vi "LSMcontroller_v59_PIzstage.vi"() -> ()   [LabVIEW 2015] (continued)
                        n2597 = Unbundle By Name(w5609) -> ("AO parameters"=w5607:T25)
                        n2598 = Index Array(array=w5607, index=0) -> (element=w5606:T26)
                        n2599 = call "generateRampedSquareWave_fromAOparameters.vi"("AO params"=w5606) -> ("Waveform"=w5602:waveform(dbl), "wflength"=w5603:i32)
                        n2600 = Build Array(w5602) -> (w5605:waveform(dbl)[])
                        n2601 = call "waveformssealtestbuffer.vi"("AO wf in"=w5605, "command"="set") -> ()  [unwired: 1 out]
                      }
                      frame #2 {
                        n2602 = local read "Vholding (mV)"() -> (w5612:sgl)
                        n2603 = local read "Current Clamp"() -> (w5618:bool)
                        n2604 = local read "Voltage Clamp"() -> (w5617:bool)
                        n2605 = local read "OCgain"() -> (w5613:sgl)
                        n2606 = local read "CC_ICgain"() -> (w5616:dbl)
                        n2607 = local read "holdon"() -> (w5611:bool)
                        n2608 = call "patchparameters.vi"("command"="get") -> ("Params out"=w5620:T14)  [unwired: 1 in]
                        n2609 = Bundle By Name(cluster=w5620, "VC"=w5617, "CC"=w5618, "CC_icg (pA/mv)"=w5616, "VC_icg (mV/mV)"=10.0, "OCG (mV/pA)"=w5613, "OVG (mV/mV)"=0.1, "Vhold (mV)"=w5612, "holdon"=w5611) -> (w5619:T14)
                        n2610 = call "patchparameters.vi"("Params in"=w5619, "command"="set") -> ()  [unwired: 1 out]
                      }
                    }
                  }
                  frame #1 {
                    w5623 = 2
                    n2611 = call "patchparameters.vi"("command"="get") -> ("Params out"=w5631:T14)  [unwired: 1 in]
                    n2612 = Unbundle By Name(w5631) -> ("holdon"=w5630:bool, "Vhold (mV)"=w5629:sgl, "CC_icg (pA/mv)"=w5637:sgl, "CC"=w5635:bool, "VC_icg (mV/mV)"=w5636:sgl)
                    n2613 = Select(t=w5637, s=w5635, f=w5636) -> (s? t:f=w5638:sgl)
                    n2614 = To Single Precision Float(number=0.001 ("y")) -> (single precision float=w5639:sgl)
                    n2615 = Compound Arithmetic op=MULTIPLY(w5629, w5638, w5639) -> (w5633:sgl)
                    n2616 = case shown="False" w5630 {
                      tunnel: w5633 -> [_ w5651]
                      tunnel: [0.0 w5651] -> w5626
                      frame False {
                      }
                      frame True {
                      }
                    }
                    n2617 = Greater Than 0?(x=w5623) -> (x > 0?=w5625:bool)
                    n2618 = case shown="True" w5625 {
                      tunnel: w5624 -> [_ w5640]
                      tunnel: w5623 -> [_ w5643]
                      frame False {
                      }
                      frame True {
                        n2619 = Initialize Array(sgl 0.0 ("element"), w5643, w5640) -> (w5641:sgl[][])
                        n2620 = call "allAI-temp.vi"("array in"=w5641, "command"=enum16{"get", "set", "clear", "append"}."set") -> ()  [unwired: 2 in, 2 out]
                      }
                    }
                    n2621 = flat-sequence {
                      tunnel: w5624 -> [w5647]
                      tunnel: w5624 -> [w5646]
                      tunnel: [w5646] -> w5628
                      tunnel: [w5645] -> w5627
                      tunnel: w5626 -> [w5645]
                      tunnel: w5628 -> [w5649]
                      tunnel: w5627 -> [w5648]
                      frame #0 {
                        n2622 = call "prepAI_sealtest.vi"("samples per channel"=w5647) -> ()  [unwired: 2 in]
                      }
                      frame #1 {
                        n2623 = call "prepAO_sealtest.vi"("Vhold"=w5648, "samples per channel"=w5649) -> ()  [unwired: 1 in]
                      }
                    }
                  }
                  frame #2 {
                    n2624 = stacked-sequence {
                      frame #0 {
                        n2625 = call "tempconfigAO.vi"("command"="get") -> ("Temp Config out"=w5655:T27)  [unwired: 1 in]
                        n2626 = Unbundle By Name(w5655) -> ("AO"=w5656:refnum<k21>[], "E_AO"=w5657:errorcluster[])
                        n2627 = for {
                          tunnel: w5656 -> [w5665] mode=indexing
                          tunnel: w5657 -> [w5664] mode=indexing
                          tunnel: [w5663] -> w5659 mode=indexing
                          tunnel: [w5662] -> w5660 mode=indexing
                          n2628 = call <vilib>:"DAQmx Start Task.vi"("task/channels in"=w5665, "error in"=w5664) -> ("task out"=w5663:refnum<k21>, "error out"=w5662:errorcluster)  [unwired: 12 in]
                        }
                        n2629 = call "tempconfigAO.vi"("command"="get") -> ("Temp Config out"=w5658:T27)  [unwired: 1 in]
                        n2630 = Bundle By Name(cluster=w5658, "AO"=w5659, "E_AO"=w5660) -> (w5661:T27)
                        n2631 = call "tempconfigAO.vi"("Temp Config in"=w5661, "command"="set") -> ()  [unwired: 1 out]
                      }
                      frame #1 {
                        n2632 = call "tempconfigAI.vi"("command"="get") -> ("Temp Config out"=w5667:T28)  [unwired: 1 in]
                        n2633 = Unbundle By Name(w5667) -> ("AI"=w5672:refnum<k21>, "E_AI"=w5673:errorcluster)
                        n2634 = call <vilib>:"DAQmx Start Task.vi"("task/channels in"=w5672, "error in"=w5673) -> ("task out"=w5674:refnum<k21>, "error out"=w5675:errorcluster)  [unwired: 12 in]
                        n2635 = call "tempconfigAI.vi"("command"="get") -> ("Temp Config out"=w5669:T28)  [unwired: 1 in]
                        n2636 = Bundle By Name(cluster=w5669, "AI"=w5674, "E_AI"=w5675) -> (w5671:T28)
                        n2637 = call "tempconfigAI.vi"("Temp Config in"=w5671, "command"="set") -> ()  [unwired: 1 out]
                      }
                    }
                  }
                  frame #3 {
                    n2638 = while {
                      tunnel: w5676 -> [w5677]
                      stop <- w5678 stop-if-true
                      n2639 = local read "sealtest"() -> (w5681:bool)
                      n2640 = Not(x=w5681) -> (.not. x?=w5680:bool)
                      n2641 = case shown="False" w5680 {
                        tunnel: w5677 -> [w5682 _]
                        frame False {
                          n2642 = stacked-sequence {
                            seq-local: [_ _ _ w5721 _ _] -> [_ _ _ _ w5777 _]
                            seq-local: [w5683 _ _ _ _ _] -> [_ w5692 _ w5714 w5766 w5797]
                            tunnel: w5682 -> [_ _ w5700 _ w5765 _]
                            frame #0 {
                              n2643 = call "patchparameters.vi"("command"="get") -> ("Params out"=w5690:T14)  [unwired: 1 in]
                              n2644 = local read "Vholding (mV)"() -> (w5687:sgl)
                              n2645 = Unbundle By Name(w5690) -> ("Vhold (mV)"=w5686:sgl, "holdon"=w5689:bool)
                              n2646 = local read "holdon"() -> (w5688:bool)
                              n2647 = Not Equal?(x=w5687, y=w5686) -> (x != y?=w5685:bool)
                              n2648 = Not Equal?(x=w5689, y=w5688) -> (x != y?=w5684:bool)
                              n2649 = Or(x=w5685, y=w5684) -> (x .or. y?=w5683:bool)
                            }
                            frame #1 {
                              n2650 = case shown="True" w5692 {
                                frame False {
                                }
                                frame True {
                                n2651 = local read "Vholding (mV)"() -> (w5695:sgl)
                                n2652 = local read "holdon"() -> (w5693:bool)
                                n2653 = call "patchparameters.vi"("command"="get") -> ("Params out"=w5696:T14)  [unwired: 1 in]
                                n2654 = Bundle By Name(cluster=w5696, "Vhold (mV)"=w5695, "holdon"=w5693) -> (w5694:T14)
                                n2655 = call "patchparameters.vi"("Params in"=w5694, "command"="set") -> ()  [unwired: 1 out]
                                }
                              }
                            }
                            frame #2 {
                              n2656 = call "tempconfigAI.vi"("command"="get") -> ("Temp Config out"=w5710:T28)  [unwired: 1 in]
                              n2657 = Unbundle By Name(w5710) -> ("AI"=w5709:refnum<k21>, "E_AI"=w5708:errorcluster)
                              n2658 = call-poly <vilib>:"DAQmx Read.vi"("task/channels in"=w5709, "number of samples per channel"=w5700, "timeout"=10.0, "error in"=w5708) -> ("task out"=w5704:refnum<k21>, "data"=w5701:i16[][], "error out"=w5713:errorcluster)  [unwired: 9 in]
                              n2659 = call "tempconfigAI.vi"("command"="get") -> ("Temp Config out"=w5705:T28)  [unwired: 1 in]
                              n2660 = Bundle By Name(cluster=w5705, "AI"=w5704, "E_AI"=w5713) -> (w5712:T28)
                              n2661 = To Single Precision Float(number=w5701) -> (single precision float=w5703:sgl[][])
                              n2662 = call "tempconfigAI.vi"("Temp Config in"=w5712, "command"="set") -> ()  [unwired: 1 out]
                              n2663 = call "allAI-temp.vi"("array in"=w5703, "command"=enum16{"get", "set", "clear", "append"}."set") -> ()  [unwired: 2 in, 2 out]
                            }
                            frame #3 {
                              n2664 = case shown="True" w5714 {
                                frame False {
                                }
                                frame True {
                                n2665 = call "tempconfigAO.vi"("command"="get") -> ("Temp Config out"=w5754:T27)  [unwired: 1 in]
                                n2666 = Unbundle By Name(w5754) -> ("AO"=w5753:refnum<k21>[], "E_AO"=w5752:errorcluster[])
                                n2667 = call "tempconfigAI.vi"("command"="get") -> ("Temp Config out"=w5741:T28)  [unwired: 1 in]
                                n2668 = Unbundle By Name(w5741) -> ("AI"=w5742:refnum<k21>, "E_AI"=w5743:errorcluster)
                                n2669 = for {
                                tunnel: w5753 -> [w5758] mode=indexing
                                tunnel: w5752 -> [w5757] mode=indexing
                                tunnel: [w5756] -> w5748 mode=indexing
                                n2670 = call <vilib>:"DAQmx Stop Task.vi"("task/channels in"=w5758, "error in"=w5757) -> ("task out"=w5759:refnum<k21>, "error out"=w5760:errorcluster)  [unwired: 12 in]
                                n2671 = call <vilib>:"DAQmx Clear Task.vi"("task in"=w5759, "error in"=w5760) -> ("error out"=w5756:errorcluster)  [unwired: 13 in]
                                }
                                n2672 = call <vilib>:"DAQmx Stop Task.vi"("task/channels in"=w5742, "error in"=w5743) -> ("task out"=w5739:refnum<k21>, "error out"=w5738:errorcluster)  [unwired: 12 in]
                                n2673 = call <vilib>:"DAQmx Clear Task.vi"("task in"=w5739, "error in"=w5738) -> ("error out"=w5737:errorcluster)  [unwired: 13 in]
                                n2674 = call "tempconfigAO.vi"("command"="get") -> ("Temp Config out"=w5749:T27)  [unwired: 1 in]
                                n2675 = Bundle By Name(cluster=w5749, "E_AO"=w5748) -> (w5747:T27)
                                n2676 = call "tempconfigAI.vi"("command"="get") -> ("Temp Config out"=w5745:T28)  [unwired: 1 in]
                                n2677 = Bundle By Name(cluster=w5745, "E_AI"=w5737) -> (w5736:T28)
                                n2678 = call "tempconfigAO.vi"("Temp Config in"=w5747, "command"="set") -> ()  [unwired: 1 out]
                                n2679 = call "tempconfigAI.vi"("Temp Config in"=w5736, "command"="set") -> ()  [unwired: 1 out]
                                }
                              }
                              n2680 = call "allAI-temp.vi"("command"=enum16{"get", "set", "clear", "append"}."get") -> ("array out"=w5718:sgl[][])  [unwired: 3 in, 1 out]
                              n2681 = call "tempconfigAI.vi"("command"="get") -> ("Temp Config out"=w5731:T28)  [unwired: 1 in]
                              n2682 = call "tempconfigAI.vi"("command"="get") -> ("Temp Config out"=w5733:T28)  [unwired: 1 in]
                              n2683 = Unbundle By Name(w5731) -> ("header"=w5729:dbl[])
                              n2684 = Unbundle By Name(w5733) -> ("header"=w5735:dbl[])
                              n2685 = Index Array(array=w5718, index (row) #1=1 ("index (row)"), index (row) #2=0 ("index (row)")) -> (element #1=w5716:sgl[], element #2=w5715:sgl[])  [unwired: 2 in]
                              n2686 = local read "OCgain"() -> (w5723:sgl)
                              n2687 = call "Unscaledtoscaled.vi"("Unscaled Data"=w5716, "Header Information"=w5729) -> ("Array"=w5728:sgl[])  [unwired: 1 in]
                              n2688 = call "Unscaledtoscaled.vi"("Unscaled Data"=w5715, "Header Information"=w5735) -> ("Array"=w5732:sgl[])  [unwired: 1 in]
                              n2689 = Multiply(x=w5728, y=0.1) -> (x*y=w5725:dbl[])
                              n2690 = Divide(x=w5732, y=w5723) -> (x/y=w5724:sgl[])
                              n2691 = Build Array(w5725, w5724) -> (w5727:dbl[][])
                              n2692 = Multiply(x=w5727, y=1000.0) -> (x*y=w5721:dbl[][])
                              "Patch readout" <- w5721
                            }
                            frame #4 {
                              n2693 = case shown="True" w5766 {
                                tunnel: w5765 -> [_ w5778]
                                frame False {
                                }
                                frame True {
                                n2694 = call "patchparameters.vi"("command"="get") -> ("Params out"=w5782:T14)  [unwired: 1 in]
                                n2695 = Unbundle By Name(w5782) -> ("holdon"=w5781:bool, "Vhold (mV)"=w5780:sgl, "CC_icg (pA/mv)"=w5788:sgl, "CC"=w5786:bool, "VC_icg (mV/mV)"=w5787:sgl)
                                n2696 = Select(t=w5788, s=w5786, f=w5787) -> (s? t:f=w5789:sgl)
                                n2697 = To Single Precision Float(number=0.001 ("y")) -> (single precision float=w5790:sgl)
                                n2698 = Compound Arithmetic op=MULTIPLY(w5780, w5789, w5790) -> (w5784:sgl)
                                n2699 = case shown="True" w5781 {
                                tunnel: w5784 -> [_ w5795]
                                tunnel: [0.0 w5795] -> w5779
                                frame False {
                                }
                                frame True {
                                }
                                }
                                n2700 = flat-sequence {
                                tunnel: w5778 -> [w5791]
                                tunnel: w5779 -> [w5793]
                                tunnel: w5778 -> [w5792]
                                frame #0 {
                                n2701 = call "prepAI_sealtest.vi"("samples per channel"=w5791) -> ()  [unwired: 2 in]
                                }
                                frame #1 {
                                n2702 = call "prepAO_sealtest.vi"("Vhold"=w5793, "samples per channel"=w5792) -> ()  [unwired: 1 in]
                                }
                                }
                                }
                              }
                              n2703 = call "sealtestwfparams.vi"("command"="get") -> ("Params out"=w5771:T24)  [unwired: 6 in]
                              n2704 = Unbundle By Name(w5771) -> ("AO parameters"=w5772:T25)
                              n2705 = Index Array(array=w5772, index=0) -> (element=w5774:T26)
                              n2706 = Unbundle By Name(w5774) -> ("Cycles"=w5769:dbl, "Start amplitude (V)"=w5768:dbl, "Sampling frequency (Hz)"=w5767:dbl)
                              n2707 = local read "fitpoints"() -> (w5775:dbl)
                              n2708 = script code="V=data(1,:);\nI=data(2,:);\ntres=mean(V);\nspc=(nsamp./ncyc);\nV=V(spc+1:end-spc);\nI=I(spc+1:end-spc);\ndV=mean(V(V>tres))-mean(V(V<tres))\nIcyc=reshape(I,[spc ncyc-2]);\nIcyc=Icyc';\nIcyc=mean(Icyc,1);\ndIss=mean(Icyc(floor(spc*0.15):floor(spc/2)-2))-mean(Icyc(spc*0.65:spc-2))\nRm=dV*1e3/dIss;\n[maxi,ind]=max(Icyc);\nIfit=Icyc(ind+1:ind+1+points-1)-0.5*(mean(Icyc(floor(spc*0.15):floor(spc/2)-2))+mean(Icyc(spc*0.65:spc-2)))\nt=(3:points-1+3)./srate*1000;\nt=t';\nIfit=Ifit';\nc=fit(t,Ifit, 'exp1');\ncoeffs=coeffvalues(c);\nIa=coeffs(1);\nRa=dV*1e3./Ia/2;\ntau=-1./coeffs(2);\ncap=tau/Ra*1000;"("data"=w5777, "nsamp"=w5765, "ncyc"=w5769, "maxV"=w5768, "points"=w5775, "srate"=w5767) -> ("cap"=w5764:dbl, "Ra"=w5763:dbl, "Icyc"=w5762:dbl[], "Rm"=w5761:dbl)  [unwired: 1 in, 1 out]
                              n2709 = local read "set as Rp?"() -> (w5776:bool)
                              n2710 = local write "Cmembrane"(w5764) -> ()
                              n2711 = local write "Rmembrane (MOhm)"(w5761) -> ()
                              n2712 = local write "Racces (MOhm)"(w5763) -> ()
                              n2713 = case shown="True" w5776 {
                                tunnel: w5761 -> [_ w5796]
                                frame False {
                                }
                                frame True {
                                n2714 = local write "Rpipette (MOhm)"(w5796) -> ()
                                }
                              }
                              n2715 = local write "Ifit"(w5762) -> ()
                            }
                            frame #5 {
                              n2716 = local read "set as Rp?"() -> (w5798:bool)
                              n2717 = case shown="True" w5797 {
                                frame False {
                                }
                                frame True {
                                n2718 = stacked-sequence {
                                frame #0 {
                                n2719 = call "tempconfigAO.vi"("command"="get") -> ("Temp Config out"=w5805:T27)  [unwired: 1 in]
                                n2720 = Unbundle By Name(w5805) -> ("AO"=w5804:refnum<k21>[], "E_AO"=w5803:errorcluster[])
                                n2721 = for {
                                tunnel: w5804 -> [w5812] mode=indexing
                                tunnel: w5803 -> [w5811] mode=indexing
                                tunnel: [w5810] -> w5801 mode=indexing
                                tunnel: [w5809] -> w5800 mode=indexing
                                n2722 = call <vilib>:"DAQmx Start Task.vi"("task/channels in"=w5812, "error in"=w5811) -> ("task out"=w5810:refnum<k21>, "error out"=w5809:errorcluster)  [unwired: 12 in]
                                }
                                n2723 = call "tempconfigAO.vi"("command"="get") -> ("Temp Config out"=w5802:T27)  [unwired: 1 in]
                                n2724 = Bundle By Name(cluster=w5802, "AO"=w5801, "E_AO"=w5800) -> (w5799:T27)
                                n2725 = call "tempconfigAO.vi"("Temp Config in"=w5799, "command"="set") -> ()  [unwired: 1 out]
                                }
                                frame #1 {
                                n2726 = call "tempconfigAI.vi"("command"="get") -> ("Temp Config out"=w5814:T28)  [unwired: 1 in]
                                n2727 = Unbundle By Name(w5814) -> ("AI"=w5819:refnum<k21>, "E_AI"=w5820:errorcluster)
                                n2728 = call <vilib>:"DAQmx Start Task.vi"("task/channels in"=w5819, "error in"=w5820) -> ("task out"=w5821:refnum<k21>, "error out"=w5822:errorcluster)  [unwired: 12 in]
                                n2729 = call "tempconfigAI.vi"("command"="get") -> ("Temp Config out"=w5816:T28)  [unwired: 1 in]
                                n2730 = Bundle By Name(cluster=w5816, "AI"=w5821, "E_AI"=w5822) -> (w5818:T28)
                                n2731 = call "tempconfigAI.vi"("Temp Config in"=w5818, "command"="set") -> ()  [unwired: 1 out]
                                }
                                }
                                }
                              }
                              n2732 = case shown="True" w5798 {
                                frame False {
                                }
                                frame True {
                                n2733 = local write "set as Rp?"(FALSE ("set as Rp?")) -> ()
                                }
                              }
                            }
                          }
                        }
                        frame True {
                        }
                      }
                      n2734 = local read "sealtest"() -> (w5679:bool)
                      n2735 = Not(x=w5679) -> (.not. x?=w5678:bool)
                    }
                  }
                  frame #4 {
                    n2736 = call "tempconfigAO.vi"("command"="get") -> ("Temp Config out"=w5849:T27)  [unwired: 1 in]
                    n2737 = Unbundle By Name(w5849) -> ("AO"=w5848:refnum<k21>[], "E_AO"=w5847:errorcluster[])
                    n2738 = call "configuration.vi"("command"="get") -> ("config out"=w5830:T12)  [unwired: 2 in, 1 out]
                    n2739 = call "tempconfigAI.vi"("command"="get") -> ("Temp Config out"=w5836:T28)  [unwired: 1 in]
                    n2740 = Unbundle By Name(w5830) -> ("Device 1 sampleclock out"=w5827:tag, "Device 1 Starttrigger out"=w5826:tag)
                    n2741 = Unbundle By Name(w5836) -> ("AI"=w5837:refnum<k21>, "E_AI"=w5838:errorcluster)
                    n2742 = for {
                      tunnel: w5848 -> [w5853] mode=indexing
                      tunnel: w5847 -> [w5852] mode=indexing
                      tunnel: [w5851] -> w5843 mode=indexing
                      n2743 = call <vilib>:"DAQmx Stop Task.vi"("task/channels in"=w5853, "error in"=w5852) -> ("task out"=w5854:refnum<k21>, "error out"=w5855:errorcluster)  [unwired: 12 in]
                      n2744 = call <vilib>:"DAQmx Clear Task.vi"("task in"=w5854, "error in"=w5855) -> ("error out"=w5851:errorcluster)  [unwired: 13 in]
                    }
                    n2745 = call <vilib>:"DAQmx Stop Task.vi"("task/channels in"=w5837, "error in"=w5838) -> ("task out"=w5834:refnum<k21>, "error out"=w5833:errorcluster)  [unwired: 12 in]
                    n2746 = call <vilib>:"DAQmx Disconnect Terminals.vi"("source terminal"=tag "/Dev1/ai/SampleClock", "destination terminal"=w5827) -> ("error out"=w5824:errorcluster)  [unwired: 13 in]
                    n2747 = call <vilib>:"DAQmx Clear Task.vi"("task in"=w5834, "error in"=w5833) -> ("error out"=w5832:errorcluster)  [unwired: 13 in]
                    n2748 = call "tempconfigAO.vi"("command"="get") -> ("Temp Config out"=w5844:T27)  [unwired: 1 in]
                    n2749 = Bundle By Name(cluster=w5844, "E_AO"=w5843) -> (w5842:T27)
                    n2750 = call "tempconfigAI.vi"("command"="get") -> ("Temp Config out"=w5840:T28)  [unwired: 1 in]
                    n2751 = Bundle By Name(cluster=w5840, "E_AI"=w5832) -> (w5831:T28)
                    n2752 = call "tempconfigAO.vi"("Temp Config in"=w5842, "command"="set") -> ()  [unwired: 1 out]
                    n2753 = call <vilib>:"DAQmx Disconnect Terminals.vi"("source terminal"=tag "/Dev1/ai/StartTrigger", "destination terminal"=w5826, "error in"=w5824) -> ()  [unwired: 12 in, 1 out]
                    n2754 = call "tempconfigAI.vi"("Temp Config in"=w5831, "command"="set") -> ()  [unwired: 1 out]
                  }
                  frame #5 {
                    w5858 = T22 4 items=["no dialog", "OK message", "continue or stop message", "OK message + warnings", "continue/stop + warnings"] ("type of dialog (OK msg:1)")
                    n2755 = call "displayerrors.vi"() -> ("error IO"=w5857:errorcluster)
                    n2756 = call "zeropatch.vi"() -> ()  [unwired: 12 in]
                    n2757 = call <vilib>:"Simple Error Handler.vi"("type of dialog (OK msg:1)"=w5858, "error in (no error)"=w5857) -> ("error out"=w5856:errorcluster)  [unwired: 3 in, 4 out]
                    n2758 = call <vilib>:"Clear Errors.vi"("error in (no error)"=w5856) -> ()  [unwired: 5 in, 2 out]
                  }
                }
              }
            }
          }
          event "readpatch": Value Change {
            n2759 = event-data() -> ()  [unwired: 1 in, 6 out]
            n2760 = local read "readpatch"() -> (w5859:bool)
            n2761 = case shown="True" w5859 {
              frame False {
              }
              frame True {
                n2762 = stacked-sequence {
                  seq-local: [w5860 _ _ _ _ _] -> [_ w5893 _ w5945 _ _]
                  frame #0 {
                    n2763 = stacked-sequence {
                      tunnel: [_ w5872 _] -> w5860
                      frame #0 {
                        n2764 = call "2pparameters.vi"("command"="get") -> ("params out"=w5865:T11)  [unwired: 1 in]
                        n2765 = Unbundle By Name(w5865) -> ("autoshutter"=w5866:bool)
                        n2766 = local read "OCchecked?"() -> (w5863:bool)
                        n2767 = call "sealtestwfparams.vi"("command"="set") -> ()  [unwired: 6 in, 1 out]
                        n2768 = case shown="False" w5863 {
                          frame False {
                            n2769 = One Button Dialog(message="Is the OC gain correct?", button name ("OK")="ok") -> (true=w5867:bool)
                            n2770 = local write "OCchecked?"(w5867) -> ()
                          }
                          frame True {
                          }
                        }
                        n2771 = case shown="True" w5866 {
                          frame False {
                          }
                          frame True {
                            n2772 = call "shuttercontrol.vi"("command"="close") -> ()  [unwired: 1 in, 1 out]
                          }
                        }
                        n2773 = call "allAI-temp.vi"("command"=enum16{"get", "set", "clear", "append"}."clear") -> ()  [unwired: 3 in, 2 out]
                      }
                      frame #1 {
                        n2774 = call "sealtestwfparams.vi"("command"="get") -> ("Params out"=w5878:T24)  [unwired: 6 in]
                        n2775 = Unbundle By Name(w5878) -> ("AO parameters"=w5876:T25)
                        n2776 = Index Array(array=w5876, index=1) -> (element=w5875:T26)
                        n2777 = call "generateRampedSquareWave_fromAOparameters.vi"("AO params"=w5875) -> ("Waveform"=w5871:waveform(dbl), "wflength"=w5872:i32)
                        n2778 = Build Array(w5871) -> (w5874:waveform(dbl)[])
                        n2779 = call "waveformssealtestbuffer.vi"("AO wf in"=w5874, "command"="set") -> ()  [unwired: 1 out]
                      }
                      frame #2 {
                        n2780 = local read "Vholding (mV)"() -> (w5881:sgl)
                        n2781 = local read "Current Clamp"() -> (w5887:bool)
                        n2782 = local read "Voltage Clamp"() -> (w5886:bool)
                        n2783 = local read "OCgain"() -> (w5882:sgl)
                        n2784 = local read "CC_ICgain"() -> (w5885:dbl)
                        n2785 = local read "holdon"() -> (w5880:bool)
                        n2786 = call "patchparameters.vi"("command"="get") -> ("Params out"=w5889:T14)  [unwired: 1 in]
                        n2787 = Bundle By Name(cluster=w5889, "VC"=w5886, "CC"=w5887, "CC_icg (pA/mv)"=w5885, "VC_icg (mV/mV)"=10.0, "OCG (mV/pA)"=w5882, "OVG (mV/mV)"=0.1, "Vhold (mV)"=w5881, "holdon"=w5880) -> (w5888:T14)
                        n2788 = call "patchparameters.vi"("Params in"=w5888, "command"="set") -> ()  [unwired: 1 out]
                      }
                    }
                  }
                  frame #1 {
                    w5892 = 2
                    n2789 = call "patchparameters.vi"("command"="get") -> ("Params out"=w5900:T14)  [unwired: 1 in]
                    n2790 = Unbundle By Name(w5900) -> ("holdon"=w5899:bool, "Vhold (mV)"=w5898:sgl, "CC_icg (pA/mv)"=w5906:sgl, "CC"=w5904:bool, "VC_icg (mV/mV)"=w5905:sgl)
                    n2791 = Select(t=w5906, s=w5904, f=w5905) -> (s? t:f=w5907:sgl)
                    n2792 = To Single Precision Float(number=0.001 ("y")) -> (single precision float=w5908:sgl)
                    n2793 = Compound Arithmetic op=MULTIPLY(w5898, w5907, w5908) -> (w5902:sgl)
                    n2794 = case shown="False" w5899 {
                      tunnel: w5902 -> [_ w5920]
                      tunnel: [0.0 w5920] -> w5895
                      frame False {
                      }
                      frame True {
                      }
                    }
                    n2795 = Greater Than 0?(x=w5892) -> (x > 0?=w5894:bool)
                    n2796 = case shown="True" w5894 {
                      tunnel: w5893 -> [_ w5909]
                      tunnel: w5892 -> [_ w5912]
                      frame False {
                      }
                      frame True {
                        n2797 = Initialize Array(sgl 0.0 ("element"), w5912, w5909) -> (w5910:sgl[][])
                        n2798 = call "allAI-temp.vi"("array in"=w5910, "command"=enum16{"get", "set", "clear", "append"}."set") -> ()  [unwired: 2 in, 2 out]
                      }
                    }
                    n2799 = flat-sequence {
                      tunnel: w5893 -> [w5916]
                      tunnel: w5893 -> [w5915]
                      tunnel: [w5915] -> w5897
                      tunnel: [w5914] -> w5896
                      tunnel: w5895 -> [w5914]
                      tunnel: w5897 -> [w5918]
                      tunnel: w5896 -> [w5917]
                      frame #0 {
                        n2800 = call "prepAI_sealtest.vi"("samples per channel"=w5916) -> ()  [unwired: 2 in]
                      }
                      frame #1 {
                        n2801 = call "prepAO_sealtest.vi"("Vhold"=w5917, "samples per channel"=w5918) -> ()  [unwired: 1 in]
                      }
                    }
                  }
                  frame #2 {
                    n2802 = stacked-sequence {
                      frame #0 {
                        n2803 = call "tempconfigAO.vi"("command"="get") -> ("Temp Config out"=w5924:T27)  [unwired: 1 in]
                        n2804 = Unbundle By Name(w5924) -> ("AO"=w5925:refnum<k21>[], "E_AO"=w5926:errorcluster[])
                        n2805 = for {
                          tunnel: w5925 -> [w5934] mode=indexing
                          tunnel: w5926 -> [w5933] mode=indexing
                          tunnel: [w5932] -> w5928 mode=indexing
                          tunnel: [w5931] -> w5929 mode=indexing
                          n2806 = call <vilib>:"DAQmx Start Task.vi"("task/channels in"=w5934, "error in"=w5933) -> ("task out"=w5932:refnum<k21>, "error out"=w5931:errorcluster)  [unwired: 12 in]
                        }
                        n2807 = call "tempconfigAO.vi"("command"="get") -> ("Temp Config out"=w5927:T27)  [unwired: 1 in]
                        n2808 = Bundle By Name(cluster=w5927, "AO"=w5928, "E_AO"=w5929) -> (w5930:T27)
                        n2809 = call "tempconfigAO.vi"("Temp Config in"=w5930, "command"="set") -> ()  [unwired: 1 out]
                      }
                      frame #1 {
                        n2810 = call "tempconfigAI.vi"("command"="get") -> ("Temp Config out"=w5936:T28)  [unwired: 1 in]
                        n2811 = Unbundle By Name(w5936) -> ("AI"=w5941:refnum<k21>, "E_AI"=w5942:errorcluster)
                        n2812 = call <vilib>:"DAQmx Start Task.vi"("task/channels in"=w5941, "error in"=w5942) -> ("task out"=w5943:refnum<k21>, "error out"=w5944:errorcluster)  [unwired: 12 in]
                        n2813 = call "tempconfigAI.vi"("command"="get") -> ("Temp Config out"=w5938:T28)  [unwired: 1 in]
                        n2814 = Bundle By Name(cluster=w5938, "AI"=w5943, "E_AI"=w5944) -> (w5940:T28)
                        n2815 = call "tempconfigAI.vi"("Temp Config in"=w5940, "command"="set") -> ()  [unwired: 1 out]
                      }
                    }
                  }
                  frame #3 {
                    n2816 = while {
                      tunnel: w5945 -> [w5946]
                      stop <- w5947 stop-if-true
                      n2817 = local read "readpatch"() -> (w5950:bool)
                      n2818 = Not(x=w5950) -> (.not. x?=w5949:bool)
                      n2819 = case shown="True" w5949 {
                        tunnel: w5946 -> [w5951 _]
                        frame False {
                          n2820 = stacked-sequence {
                            seq-local: [w5952 _ _ _ _ _] -> [_ w5961 _ w5984 w6031 w6050]
                            tunnel: w5951 -> [_ _ w5969 _ w6030 _]
                            frame #0 {
                              n2821 = call "patchparameters.vi"("command"="get") -> ("Params out"=w5959:T14)  [unwired: 1 in]
                              n2822 = local read "Vholding (mV)"() -> (w5956:sgl)
                              n2823 = Unbundle By Name(w5959) -> ("Vhold (mV)"=w5955:sgl, "holdon"=w5958:bool)
                              n2824 = local read "holdon"() -> (w5957:bool)
                              n2825 = Not Equal?(x=w5956, y=w5955) -> (x != y?=w5954:bool)
                              n2826 = Not Equal?(x=w5958, y=w5957) -> (x != y?=w5953:bool)
                              n2827 = Or(x=w5954, y=w5953) -> (x .or. y?=w5952:bool)
                            }
                            frame #1 {
                              n2828 = case shown="False" w5961 {
                                frame False {
                                }
                                frame True {
                                n2829 = local read "Vholding (mV)"() -> (w5964:sgl)
                                n2830 = local read "holdon"() -> (w5962:bool)
                                n2831 = call "patchparameters.vi"("command"="get") -> ("Params out"=w5965:T14)  [unwired: 1 in]
                                n2832 = Bundle By Name(cluster=w5965, "Vhold (mV)"=w5964, "holdon"=w5962) -> (w5963:T14)
                                n2833 = call "patchparameters.vi"("Params in"=w5963, "command"="set") -> ()  [unwired: 1 out]
                                }
                              }
                            }
                            frame #2 {
                              n2834 = call "tempconfigAI.vi"("command"="get") -> ("Temp Config out"=w5979:T28)  [unwired: 1 in]
                              n2835 = Unbundle By Name(w5979) -> ("AI"=w5978:refnum<k21>, "E_AI"=w5977:errorcluster)
                              n2836 = call-poly <vilib>:"DAQmx Read.vi"("task/channels in"=w5978, "number of samples per channel"=w5969, "timeout"=10.0, "error in"=w5977) -> ("task out"=w5973:refnum<k21>, "data"=w5970:i16[][], "error out"=w5982:errorcluster)  [unwired: 9 in]
                              n2837 = call "tempconfigAI.vi"("command"="get") -> ("Temp Config out"=w5974:T28)  [unwired: 1 in]
                              n2838 = Bundle By Name(cluster=w5974, "AI"=w5973, "E_AI"=w5982) -> (w5981:T28)
                              n2839 = To Single Precision Float(number=w5970) -> (single precision float=w5972:sgl[][])
                              n2840 = call "tempconfigAI.vi"("Temp Config in"=w5981, "command"="set") -> ()  [unwired: 1 out]
                              n2841 = call "allAI-temp.vi"("array in"=w5972, "command"=enum16{"get", "set", "clear", "append"}."set") -> ()  [unwired: 2 in, 2 out]
                            }
                            frame #3 {
                              n2842 = case shown="True" w5984 {
                                frame False {
                                }
                                frame True {
                                n2843 = call "tempconfigAO.vi"("command"="get") -> ("Temp Config out"=w6023:T27)  [unwired: 1 in]
                                n2844 = Unbundle By Name(w6023) -> ("AO"=w6022:refnum<k21>[], "E_AO"=w6021:errorcluster[])
                                n2845 = call "tempconfigAI.vi"("command"="get") -> ("Temp Config out"=w6010:T28)  [unwired: 1 in]
                                n2846 = Unbundle By Name(w6010) -> ("AI"=w6011:refnum<k21>, "E_AI"=w6012:errorcluster)
                                n2847 = for {
                                tunnel: w6022 -> [w6027] mode=indexing
                                tunnel: w6021 -> [w6026] mode=indexing
                                tunnel: [w6025] -> w6017 mode=indexing
                                n2848 = call <vilib>:"DAQmx Stop Task.vi"("task/channels in"=w6027, "error in"=w6026) -> ("task out"=w6028:refnum<k21>, "error out"=w6029:errorcluster)  [unwired: 12 in]
                                n2849 = call <vilib>:"DAQmx Clear Task.vi"("task in"=w6028, "error in"=w6029) -> ("error out"=w6025:errorcluster)  [unwired: 13 in]
                                }
                                n2850 = call <vilib>:"DAQmx Stop Task.vi"("task/channels in"=w6011, "error in"=w6012) -> ("task out"=w6008:refnum<k21>, "error out"=w6007:errorcluster)  [unwired: 12 in]
                                n2851 = call <vilib>:"DAQmx Clear Task.vi"("task in"=w6008, "error in"=w6007) -> ("error out"=w6006:errorcluster)  [unwired: 13 in]
                                n2852 = call "tempconfigAO.vi"("command"="get") -> ("Temp Config out"=w6018:T27)  [unwired: 1 in]
                                n2853 = Bundle By Name(cluster=w6018, "E_AO"=w6017) -> (w6016:T27)
                                n2854 = call "tempconfigAI.vi"("command"="get") -> ("Temp Config out"=w6014:T28)  [unwired: 1 in]
                                n2855 = Bundle By Name(cluster=w6014, "E_AI"=w6006) -> (w6005:T28)
                                n2856 = call "tempconfigAO.vi"("Temp Config in"=w6016, "command"="set") -> ()  [unwired: 1 out]
                                n2857 = call "tempconfigAI.vi"("Temp Config in"=w6005, "command"="set") -> ()  [unwired: 1 out]
                                }
                              }
                              n2858 = call "allAI-temp.vi"("command"=enum16{"get", "set", "clear", "append"}."get") -> ("array out"=w5988:sgl[][])  [unwired: 3 in, 1 out]
                              n2859 = call "tempconfigAI.vi"("command"="get") -> ("Temp Config out"=w6000:T28)  [unwired: 1 in]
                              n2860 = call "tempconfigAI.vi"("command"="get") -> ("Temp Config out"=w6002:T28)  [unwired: 1 in]
                              n2861 = Unbundle By Name(w6000) -> ("header"=w5998:dbl[])
                              n2862 = Unbundle By Name(w6002) -> ("header"=w6004:dbl[])
                              n2863 = Index Array(array=w5988, index (row) #1=1 ("index (row)"), index (row) #2=0 ("index (row)")) -> (element #1=w5986:sgl[], element #2=w5985:sgl[])  [unwired: 2 in]
                              n2864 = local read "OCgain"() -> (w5992:sgl)
                              n2865 = call "Unscaledtoscaled.vi"("Unscaled Data"=w5986, "Header Information"=w5998) -> ("Array"=w5997:sgl[])  [unwired: 1 in]
                              n2866 = call "Unscaledtoscaled.vi"("Unscaled Data"=w5985, "Header Information"=w6004) -> ("Array"=w6001:sgl[])  [unwired: 1 in]
                              n2867 = Multiply(x=w5997, y=0.1) -> (x*y=w5994:dbl[])
                              n2868 = Divide(x=w6001, y=w5992) -> (x/y=w5993:sgl[])
                              n2869 = Build Array(w5994, w5993) -> (w5996:dbl[][])
                              n2870 = Multiply(x=w5996, y=1000.0) -> (x*y=w5983:dbl[][])
                              n2871 = local write "Patch readout"(w5983) -> ()
                            }
                            frame #4 {
                              n2872 = case shown="True" w6031 {
                                tunnel: w6030 -> [_ w6032]
                                frame False {
                                }
                                frame True {
                                n2873 = call "patchparameters.vi"("command"="get") -> ("Params out"=w6036:T14)  [unwired: 1 in]
                                n2874 = Unbundle By Name(w6036) -> ("holdon"=w6035:bool, "Vhold (mV)"=w6034:sgl, "CC_icg (pA/mv)"=w6042:sgl, "CC"=w6040:bool, "VC_icg (mV/mV)"=w6041:sgl)
                                n2875 = Select(t=w6042, s=w6040, f=w6041) -> (s? t:f=w6043:sgl)
                                n2876 = To Single Precision Float(number=0.001 ("y")) -> (single precision float=w6044:sgl)
                                n2877 = Compound Arithmetic op=MULTIPLY(w6034, w6043, w6044) -> (w6038:sgl)
                                n2878 = case shown="True" w6035 {
                                tunnel: w6038 -> [_ w6049]
                                tunnel: [0.0 w6049] -> w6033
                                frame False {
                                }
                                frame True {
                                }
                                }
                                n2879 = flat-sequence {
                                tunnel: w6032 -> [w6045]
                                tunnel: w6033 -> [w6047]
                                tunnel: w6032 -> [w6046]
                                frame #0 {
                                n2880 = call "prepAI_sealtest.vi"("samples per channel"=w6045) -> ()  [unwired: 2 in]
                                }
                                frame #1 {
                                n2881 = call "prepAO_sealtest.vi"("Vhold"=w6047, "samples per channel"=w6046) -> ()  [unwired: 1 in]
                                }
                                }
                                }
                              }
                            }
                            frame #5 {
                              n2882 = case shown="True" w6050 {
                                frame False {
                                }
                                frame True {
                                n2883 = stacked-sequence {
                                frame #0 {
                                n2884 = call "tempconfigAO.vi"("command"="get") -> ("Temp Config out"=w6057:T27)  [unwired: 1 in]
                                n2885 = Unbundle By Name(w6057) -> ("AO"=w6056:refnum<k21>[], "E_AO"=w6055:errorcluster[])
                                n2886 = for {
                                tunnel: w6056 -> [w6064] mode=indexing
                                tunnel: w6055 -> [w6063] mode=indexing
                                tunnel: [w6062] -> w6053 mode=indexing
                                tunnel: [w6061] -> w6052 mode=indexing
                                n2887 = call <vilib>:"DAQmx Start Task.vi"("task/channels in"=w6064, "error in"=w6063) -> ("task out"=w6062:refnum<k21>, "error out"=w6061:errorcluster)  [unwired: 12 in]
                                }
                                n2888 = call "tempconfigAO.vi"("command"="get") -> ("Temp Config out"=w6054:T27)  [unwired: 1 in]
                                n2889 = Bundle By Name(cluster=w6054, "AO"=w6053, "E_AO"=w6052) -> (w6051:T27)
                                n2890 = call "tempconfigAO.vi"("Temp Config in"=w6051, "command"="set") -> ()  [unwired: 1 out]
                                }
                                frame #1 {
                                n2891 = call "tempconfigAI.vi"("command"="get") -> ("Temp Config out"=w6066:T28)  [unwired: 1 in]
                                n2892 = Unbundle By Name(w6066) -> ("AI"=w6071:refnum<k21>, "E_AI"=w6072:errorcluster)
                                n2893 = call <vilib>:"DAQmx Start Task.vi"("task/channels in"=w6071, "error in"=w6072) -> ("task out"=w6073:refnum<k21>, "error out"=w6074:errorcluster)  [unwired: 12 in]
                                n2894 = call "tempconfigAI.vi"("command"="get") -> ("Temp Config out"=w6068:T28)  [unwired: 1 in]
                                n2895 = Bundle By Name(cluster=w6068, "AI"=w6073, "E_AI"=w6074) -> (w6070:T28)
                                n2896 = call "tempconfigAI.vi"("Temp Config in"=w6070, "command"="set") -> ()  [unwired: 1 out]
                                }
                                }
                                }
                              }
                            }
                          }
                        }
                        frame True {
                        }
                      }
                      n2897 = local read "readpatch"() -> (w5948:bool)
                      n2898 = Not(x=w5948) -> (.not. x?=w5947:bool)
                    }
                  }
                  frame #4 {
                    n2899 = call "tempconfigAO.vi"("command"="get") -> ("Temp Config out"=w6100:T27)  [unwired: 1 in]
                    n2900 = Unbundle By Name(w6100) -> ("AO"=w6099:refnum<k21>[], "E_AO"=w6098:errorcluster[])
                    n2901 = call "configuration.vi"("command"="get") -> ("config out"=w6081:T12)  [unwired: 2 in, 1 out]
                    n2902 = call "tempconfigAI.vi"("command"="get") -> ("Temp Config out"=w6087:T28)  [unwired: 1 in]
                    n2903 = Unbundle By Name(w6081) -> ("Device 1 sampleclock out"=w6078:tag, "Device 1 Starttrigger out"=w6077:tag)
                    n2904 = Unbundle By Name(w6087) -> ("AI"=w6088:refnum<k21>, "E_AI"=w6089:errorcluster)
                    n2905 = for {
                      tunnel: w6099 -> [w6104] mode=indexing
                      tunnel: w6098 -> [w6103] mode=indexing
                      tunnel: [w6102] -> w6094 mode=indexing
                      n2906 = call <vilib>:"DAQmx Stop Task.vi"("task/channels in"=w6104, "error in"=w6103) -> ("task out"=w6105:refnum<k21>, "error out"=w6106:errorcluster)  [unwired: 12 in]
                      n2907 = call <vilib>:"DAQmx Clear Task.vi"("task in"=w6105, "error in"=w6106) -> ("error out"=w6102:errorcluster)  [unwired: 13 in]
                    }
                    n2908 = call <vilib>:"DAQmx Stop Task.vi"("task/channels in"=w6088, "error in"=w6089) -> ("task out"=w6085:refnum<k21>, "error out"=w6084:errorcluster)  [unwired: 12 in]
                    n2909 = call <vilib>:"DAQmx Disconnect Terminals.vi"("source terminal"=tag "/Dev1/ai/SampleClock", "destination terminal"=w6078) -> ("error out"=w6075:errorcluster)  [unwired: 13 in]
                    n2910 = call <vilib>:"DAQmx Clear Task.vi"("task in"=w6085, "error in"=w6084) -> ("error out"=w6083:errorcluster)  [unwired: 13 in]
                    n2911 = call "tempconfigAO.vi"("command"="get") -> ("Temp Config out"=w6095:T27)  [unwired: 1 in]
                    n2912 = Bundle By Name(cluster=w6095, "E_AO"=w6094) -> (w6093:T27)
                    n2913 = call "tempconfigAI.vi"("command"="get") -> ("Temp Config out"=w6091:T28)  [unwired: 1 in]
                    n2914 = Bundle By Name(cluster=w6091, "E_AI"=w6083) -> (w6082:T28)
                    n2915 = call "tempconfigAO.vi"("Temp Config in"=w6093, "command"="set") -> ()  [unwired: 1 out]
                    n2916 = call <vilib>:"DAQmx Disconnect Terminals.vi"("source terminal"=tag "/Dev1/ai/StartTrigger", "destination terminal"=w6077, "error in"=w6075) -> ()  [unwired: 12 in, 1 out]
                    n2917 = call "tempconfigAI.vi"("Temp Config in"=w6082, "command"="set") -> ()  [unwired: 1 out]
                  }
                  frame #5 {
                    w6109 = T22 4 items=["no dialog", "OK message", "continue or stop message", "OK message + warnings", "continue/stop + warnings"] ("type of dialog (OK msg:1)")
                    n2918 = call "displayerrors.vi"() -> ("error IO"=w6108:errorcluster)
                    n2919 = call "zeropatch.vi"() -> ()  [unwired: 12 in]
                    n2920 = call <vilib>:"Simple Error Handler.vi"("type of dialog (OK msg:1)"=w6109, "error in (no error)"=w6108) -> ("error out"=w6107:errorcluster)  [unwired: 3 in, 4 out]
                    n2921 = call <vilib>:"Clear Errors.vi"("error in (no error)"=w6107) -> ()  [unwired: 5 in, 2 out]
                  }
                }
              }
            }
          }
          event "Current Clamp": Value Change {
            n2922 = event-data() -> ()  [unwired: 1 in, 6 out]
            n2923 = local read "Current Clamp"() -> (w6114:bool)
            n2924 = property on="Vholding (mV)" class="DigNum (strict)"("Caption.Text"="Ihold (pA)") -> ()  [unwired: 2 in, 2 out]
            n2925 = Not(x=w6114) -> (.not. x?=w6113:bool)
            n2926 = property on="Voltage Clamp" class="Bool (strict)"("Value"=w6113) -> ()  [unwired: 2 in, 2 out]
            n2927 = One Button Dialog(message="Have you switched the HEKA to CC and changed the external input cable?", button name ("OK")="Ok") -> ()  [unwired: 1 out]
          }
          event "Voltage Clamp": Value Change {
            n2928 = event-data() -> ()  [unwired: 1 in, 6 out]
            n2929 = local read "Voltage Clamp"() -> (w6119:bool)
            n2930 = Not(x=w6119) -> (.not. x?=w6118:bool)
            n2931 = property on="Current Clamp" class="Bool (strict)"("Value"=w6118) -> ()  [unwired: 2 in, 2 out]
            n2932 = One Button Dialog(message="Have you switched the HEKA to VC and changed the external input cable?", button name ("OK")="Ok") -> ()  [unwired: 1 out]
            n2933 = property on="Vholding (mV)" class="DigNum (strict)"("Caption.Text"="Vhold (mV)") -> ()  [unwired: 2 in, 2 out]
          }
          event "OCgain": Value Change {
            n2934 = event-data() -> ()  [unwired: 1 in, 6 out]
            n2935 = local read "OCgain"() -> (w6122:sgl)
            n2936 = Less?(x=w6122, y=0.3) -> (x < y?=w6120:bool)
            n2937 = case shown="True" w6120 {
              frame False {
                w6123 = 10.0 items=["0.1"=10.0, "10"=0.1] ("CC_ICgain")
                n2938 = local write "CC_ICgain"(w6123) -> ()
              }
              frame True {
                w6124 = 0.1 items=["0.1"=10.0, "10"=0.1] ("CC_ICgain")
                n2939 = local write "CC_ICgain"(w6124) -> ()
              }
            }
          }
          event "holdon": Value Change {
            n2940 = event-data() -> ()  [unwired: 1 in, 6 out]
            n2941 = stacked-sequence {
              frame #0 {
                n2942 = local read "Vholding (mV)"() -> (w6128:sgl)
                n2943 = local read "holdon"() -> (w6125:bool)
                n2944 = call "patchparameters.vi"("command"="get") -> ("Params out"=w6129:T14)  [unwired: 1 in]
                n2945 = Bundle By Name(cluster=w6129, "Vhold (mV)"=w6128, "holdon"=w6125) -> (w6126:T14)
                n2946 = call "patchparameters.vi"("Params in"=w6126, "command"="set") -> ()  [unwired: 1 out]
              }
              frame #1 {
                n2947 = call "zeropatch.vi"() -> ()  [unwired: 12 in]
              }
            }
          }
          event "Vholding (mV)": Value Change {
            n2948 = event-data() -> ()  [unwired: 1 in, 6 out]
            n2949 = local read "holdon"() -> (w6131:bool)
            n2950 = case shown="True" w6131 {
              frame False {
              }
              frame True {
                n2951 = stacked-sequence {
                  frame #0 {
                    n2952 = local read "Vholding (mV)"() -> (w6134:sgl)
                    n2953 = local read "holdon"() -> (w6135:bool)
                    n2954 = call "patchparameters.vi"("command"="get") -> ("Params out"=w6136:T14)  [unwired: 1 in]
                    n2955 = Bundle By Name(cluster=w6136, "Vhold (mV)"=w6134, "holdon"=w6135) -> (w6132:T14)
                    n2956 = call "patchparameters.vi"("Params in"=w6132, "command"="set") -> ()  [unwired: 1 out]
                  }
                  frame #1 {
                    n2957 = call "zeropatch.vi"() -> ()  [unwired: 12 in]
                  }
                }
              }
            }
          }
          event "AI channels": Value Change {
            n2958 = event-data() -> ()  [unwired: 1 in, 6 out]
            n2959 = local read "CI channels"() -> (w6145:i32[])
            n2960 = local read "AI channels"() -> (w6146:i32[])
            n2961 = call "configuration.vi"("command"="get") -> ("config out"=w6139:T12)  [unwired: 2 in, 1 out]
            n2962 = Unbundle By Name(w6139) -> ("CI names"=w6140:string[], "AI names"=w6141:string[])
            n2963 = for {
              tunnel: w6145 -> [w6151] mode=indexing
              tunnel: w6140 -> [w6152]
              tunnel: [w6150] -> w6142 mode=indexing
              n2964 = Index Array(array=w6152, index=w6151) -> (element=w6150:string)
            }
            n2965 = for {
              tunnel: w6146 -> [w6148] mode=indexing
              tunnel: w6141 -> [w6149]
              tunnel: [w6147] -> w6143 mode=indexing
              n2966 = Index Array(array=w6149, index=w6148) -> (element=w6147:string)
            }
            n2967 = Build Array (concatenate)(w6142, w6143) -> (w6144:string[])
            n2968 = property on="image1list" class="Ring (strict)"("Strings []"=w6144) -> ()  [unwired: 2 in, 2 out]
            n2969 = property on="image2list" class="Ring (strict)"("Strings []"=w6144) -> ()  [unwired: 2 in, 2 out]
          }
          event "CI channels": Value Change {
            n2970 = event-data() -> ()  [unwired: 1 in, 6 out]
            n2971 = local read "CI channels"() -> (w6160:i32[])
            n2972 = local read "AI channels"() -> (w6161:i32[])
            n2973 = call "configuration.vi"("command"="get") -> ("config out"=w6154:T12)  [unwired: 2 in, 1 out]
            n2974 = Unbundle By Name(w6154) -> ("CI names"=w6155:string[], "AI names"=w6156:string[])
            n2975 = for {
              tunnel: w6160 -> [w6166] mode=indexing
              tunnel: w6155 -> [w6167]
              tunnel: [w6165] -> w6157 mode=indexing
              n2976 = Index Array(array=w6167, index=w6166) -> (element=w6165:string)
            }
            n2977 = for {
              tunnel: w6161 -> [w6163] mode=indexing
              tunnel: w6156 -> [w6164]
              tunnel: [w6162] -> w6158 mode=indexing
              n2978 = Index Array(array=w6164, index=w6163) -> (element=w6162:string)
            }
            n2979 = Build Array (concatenate)(w6157, w6158) -> (w6159:string[])
            n2980 = property on="image1list" class="Ring (strict)"("Strings []"=w6159) -> ()  [unwired: 2 in, 2 out]
            n2981 = property on="image2list" class="Ring (strict)"("Strings []"=w6159) -> ()  [unwired: 2 in, 2 out]
          }
          event "setdatdir": Value Change {
            n2982 = event-data() -> ()  [unwired: 1 in, 5 out]
            n2983 = case shown="True" "setdatdir" {
              frame False {
              }
              frame True {
                n2984 = stacked-sequence {
                  frame #0 {
                    n2985 = local read "data dir"() -> (w6169:path)
                    n2986 = call "File Dialog"("start path"=w6169, "prompt"="Please select data directory...") -> ("selected path"=w6171:path, "cancelled"=w6170:bool, "error out"=w6172:errorcluster)  [unwired: 10 in, 1 out]
                    n2987 = case shown="False" w6170 {
                      tunnel: w6171 -> [w6180 _]
                      tunnel: w6172 -> [w6177 w6183]
                      tunnel: [w6175 w6183] -> w6174
                      frame False {
                        n2988 = local write "data dir"(w6180) -> ()
                        n2989 = call "configuration.vi"("error in"=w6177, "command"="get") -> ("Error out"=w6176:errorcluster, "config out"=w6182:T12)  [unwired: 1 in]
                        n2990 = Bundle By Name(cluster=w6182, "master data dir"=w6180) -> (w6181:T12)
                        n2991 = call "configuration.vi"("error in"=w6176, "config in"=w6181, "command"="set") -> ("Error out"=w6175:errorcluster)  [unwired: 1 out]
                      }
                      frame True {
                      }
                    }
                    n2992 = local write "status"(w6174) -> ()
                  }
                  frame #1 {
                    n2993 = property on="setdatdir" class="Bool (strict)"("Value"=FALSE ("setdatdir")) -> ()  [unwired: 2 in, 2 out]
                  }
                }
              }
            }
          }
          event "Shutter": Value Change {
            n2994 = event-data() -> ()  [unwired: 1 in, 5 out]
            n2995 = case shown="False" "Shutter" {
              frame False {
                n2996 = call "shuttercontrol.vi"("command"="close") -> ()  [unwired: 1 in, 1 out]
              }
              frame True {
                n2997 = call "shuttercontrol.vi"("command"="open") -> ()  [unwired: 1 in, 1 out]
              }
            }
          }
          event "ROI": Value Change {
            n2998 = event-data() -> ()  [unwired: 1 in, 5 out]
            n2999 = local read "ROI"() -> (w6188:bool)
            n3000 = case shown="True" w6188 {
              frame False {
              }
              frame True {
                n3001 = stacked-sequence {
                  frame #0 {
                    n3002 = local read "Square pixels"() -> (w6205:bool)
                    n3003 = local read "square matrix"() -> (w6204:bool)
                    n3004 = local read "Vx-max ref"() -> (w6210:dbl)
                    n3005 = local read "Vx-min ref"() -> (w6209:dbl)
                    n3006 = local read "Vy-min ref"() -> (w6206:dbl)
                    n3007 = local read "ypixels ref"() -> (w6208:i32)
                    n3008 = local read "Vy-max ref"() -> (w6207:dbl)
                    n3009 = local read "xpixels ref"() -> (w6211:i32)
                    n3010 = local read "Angle ref"() -> (w6203:dbl)
                    n3011 = local read "Colormap"() -> (w6212:i32)
                    n3012 = call "2pparameters.vi"("command"="get") -> ("params out"=w6215:T11)  [unwired: 1 in]
                    n3013 = Bundle By Name(cluster=w6215, "Xpixels Img"=w6211, "Vx-min Img"=w6209, "VX-max Img"=w6210, "Ypixels Img"=w6208, "Vy-min Img"=w6206, "Vy-max Img"=w6207, "Colormap"=w6212, "square pixels"=w6205, "square matrix"=w6204, "Angle Img"=w6203) -> (w6214:T11)
                    n3014 = call "2pparameters.vi"("Params in"=w6214, "command"="set") -> ()  [unwired: 1 out]
                    n3015 = local read "Vx-max draw"() -> (w6195:dbl)
                    n3016 = local read "Angle drawing"() -> (w6202:dbl)
                    n3017 = local read "Vx-min draw"() -> (w6196:dbl)
                    n3018 = local read "Vy-min draw"() -> (w6199:dbl)
                    n3019 = local read "ypixels draw"() -> (w6197:dbl)
                    n3020 = local read "Vy-max draw"() -> (w6198:dbl)
                    n3021 = local read "Square pixels"() -> (w6200:bool)
                    n3022 = local read "square matrix"() -> (w6201:bool)
                    n3023 = local read "xpixels draw"() -> (w6194:dbl)
                    n3024 = local read "Colormap"() -> (w6193:i32)
                    n3025 = call "2pparameters.vi"("command"="get") -> ("params out"=w6190:T11)  [unwired: 1 in]
                    n3026 = Bundle By Name(cluster=w6190, "Xpixels"=w6194, "Vxminref"=w6196, "Vxmaxref"=w6195, "Ypixels"=w6197, "Vyminref"=w6199, "Vymaxref"=w6198, "Colormap"=w6193, "square pixels"=w6200, "square matrix"=w6201, "Angle draw"=w6202) -> (w6191:T11)
                    n3027 = call "2pparameters.vi"("Params in"=w6191, "command"="set") -> ()  [unwired: 1 out]
                  }
                  frame #1 {
                    n3028 = Current VI's Path() -> (path=w6226:path)
                    n3029 = Strip Path(path=w6226) -> (stripped path=w6227:path)  [unwired: 1 out]
                    n3030 = Build Path(base path=w6227, name or relative path="subVIs\\Image\\SetROI_v3.vi") -> (appended path=w6225:path)
                    n3031 = call <vilib>:"Set Busy.vi"() -> ("error out"=w6223:errorcluster)  [unwired: 10 in, 1 out]
                    n3032 = Open VI Reference(type specifier VI Refnum (for type only)=refnum<vi> refnum, vi path=w6225, error in (no error)=w6223) -> (vi reference=w6221:refnum<vi>, error out=w6219:errorcluster)  [unwired: 3 in]
                    n3033 = call-by-ref "?"(reference=w6221, error in=w6219) -> (reference out=w6220:refnum<vi>, error out=w6218:errorcluster)  [unwired: 1 in]
                    n3034 = Close Reference(reference=w6220, error in (no error)=w6218) -> (error out=w6222:errorcluster)
                    n3035 = call <vilib>:"Unset Busy.vi"("error in (no error)"=w6222) -> ()  [unwired: 10 in, 1 out]
                    n3036 = local write "status"(w6222) -> ()
                  }
                  frame #2 {
                    n3037 = call "2pparameters.vi"("command"="get") -> ("params out"=w6252:T11)  [unwired: 1 in]
                    n3038 = Unbundle By Name(w6252) -> ("Xpixels Img"=w6251:i32, "Vx-min Img"=w6250:dbl, "VX-max Img"=w6249:dbl, "Ypixels Img"=w6248:i32, "Vy-min Img"=w6247:dbl, "Vy-max Img"=w6246:dbl, "Colormap"=w6245:u16, "square pixels"=w6244:bool, "square matrix"=w6243:bool, "Angle Img"=w6242:dbl, "Drawing Mode"=w6241:u16)
                    n3039 = local write "xpixels ref"(w6251) -> ()
                    n3040 = local write "Vx-min ref"(w6250) -> ()
                    n3041 = local write "Vx-max ref"(w6249) -> ()
                    n3042 = local write "ypixels ref"(w6248) -> ()
                    n3043 = local write "Vy-min ref"(w6247) -> ()
                    n3044 = local write "Vy-max ref"(w6246) -> ()
                    n3045 = local write "Colormap"(w6245) -> ()
                    n3046 = local write "Square pixels"(w6244) -> ()
                    n3047 = local write "square matrix"(w6243) -> ()
                    n3048 = local write "Angle ref"(w6242) -> ()
                    n3049 = local write "ROI Type"(w6241) -> ()
                    n3050 = call "2pparameters.vi"("command"="get") -> ("params out"=w6235:T11)  [unwired: 1 in]
                    n3051 = Unbundle By Name(w6235) -> ("Xpixels"=w6229:i32, "Vxminref"=w6233:dbl, "Vxmaxref"=w6232:dbl, "Ypixels"=w6228:i32, "Vyminref"=w6231:dbl, "Vymaxref"=w6230:dbl, "Colormap"=w6236:u16, "square pixels"=w6237:bool, "square matrix"=w6238:bool, "Angle draw"=w6239:dbl, "Drawing Mode"=w6240:u16)
                    n3052 = local write "Vy-max draw"(w6230) -> ()
                    n3053 = local write "Angle drawing"(w6239) -> ()
                    n3054 = local write "Colormap"(w6236) -> ()
                    n3055 = local write "Square pixels"(w6237) -> ()
                    n3056 = local write "square matrix"(w6238) -> ()
                    n3057 = local write "ROI Type"(w6240) -> ()
                    n3058 = local write "xpixels draw"(w6229) -> ()
                    n3059 = local write "ypixels draw"(w6228) -> ()
                    n3060 = local write "Vx-min draw"(w6233) -> ()
                    n3061 = local write "Vx-max draw"(w6232) -> ()
                    n3062 = local write "Vy-min draw"(w6231) -> ()
                  }
                  frame #3 {
